vi "1.4.vi"() -> ()   [LabVIEW 2016]
panel:
  in  "度数":dbl
  out "弧度":dbl format="%#_3g"
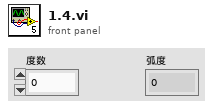
[diagram p1: front panel]
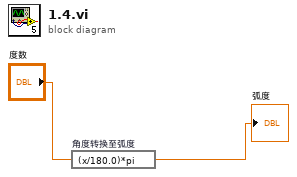
[diagram p0: block diagram]
diagram:
  n1 = expression code="(x/180.0)*pi" "角度转换至弧度"("度数") -> (→"弧度":dbl)
